vi "Test Symmetric (DBL).vi"(9 "relative tolerance?":bool, 10 "tolerance":dbl=-1.0, 11 "Input Matrix":T1) -> (0 "error":i32, 3 "symmetric?":bool)   [LabVIEW 2010, in "NI_AALPro.lvlib"]
uses:
  NI_AALPro.lvlib
  RealMatrix.ctl
  lvanlys.dll
  NI_Matrix.lvlib
panel:
  # "Test Symmetric"
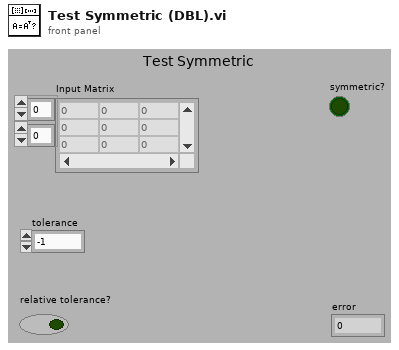
[diagram p1: front panel]
types:
  T1 = typedef "NI_Matrix.lvlib/RealMatrix.ctl" = dbl[][]
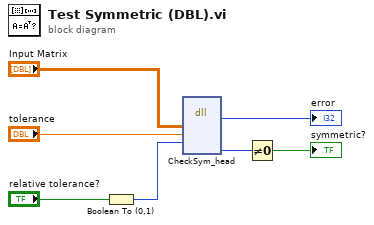
[diagram p0: block diagram]
diagram:
  n1 = Boolean To (0,1)(Boolean="relative tolerance?") -> (0, 1=w2:i16)
  n2 = dll-call lib="C:/Program Files/National Instruments/LabVIEW 2010/resource/lvanlys.*" fn="CheckSym_head" ("lvanlys.dll:CheckPosSemiDef_head")("_aH"="Input Matrix", "_tol"="tolerance", "_reltol"=w2) -> ("return type"=→"error":i32, "_sym"=w5:i32)  [unwired: 5 in, 4 out]
  n3 = Not Equal To 0?(x=w5) -> (x != 0?=→"symmetric?":bool)
